vi "getFATimestamp.vi"(11 "ILCCommunications in":refnum<class "ILCCommunications.lvclass">) -> (2 "FATimestamp":T1, 3 "ILCCommunications out":refnum<class "ILCCommunications.lvclass">)   [LabVIEW 2016, in "ILCCommunications.lvclass"]
uses:
  ILCCommunications.lvclass
  DataTypes/Topics/Parts/Timestamp.ctl
  ILCCommunications.lvclass/ILCCommunications.ctl
  DataTypes/Topics/M1M3SupportTopics.lvlib
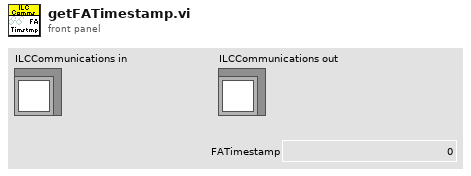
[diagram p1: front panel]
types:
  T1 = typedef "M1M3SupportTopics.lvlib/Timestamp.ctl" = dbl
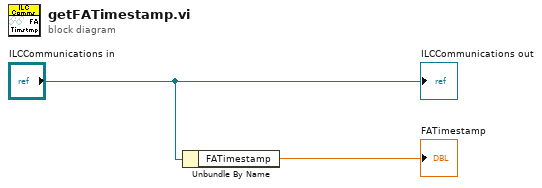
[diagram p0: block diagram]
diagram:
  n1 = Unbundle By Name("ILCCommunications in") -> ("FATimestamp"=→"FATimestamp":T1)
  "ILCCommunications out" <- "ILCCommunications in"
